vi "校准信息转u16数组.vi"(11 "关键参数":T1(array[cluster])) -> (3 "添加的数组":u16[](array[numeric]))   [LabVIEW 2016, in "MB SLAVE.lvlib"]
uses:
  MB SLAVE.lvlib
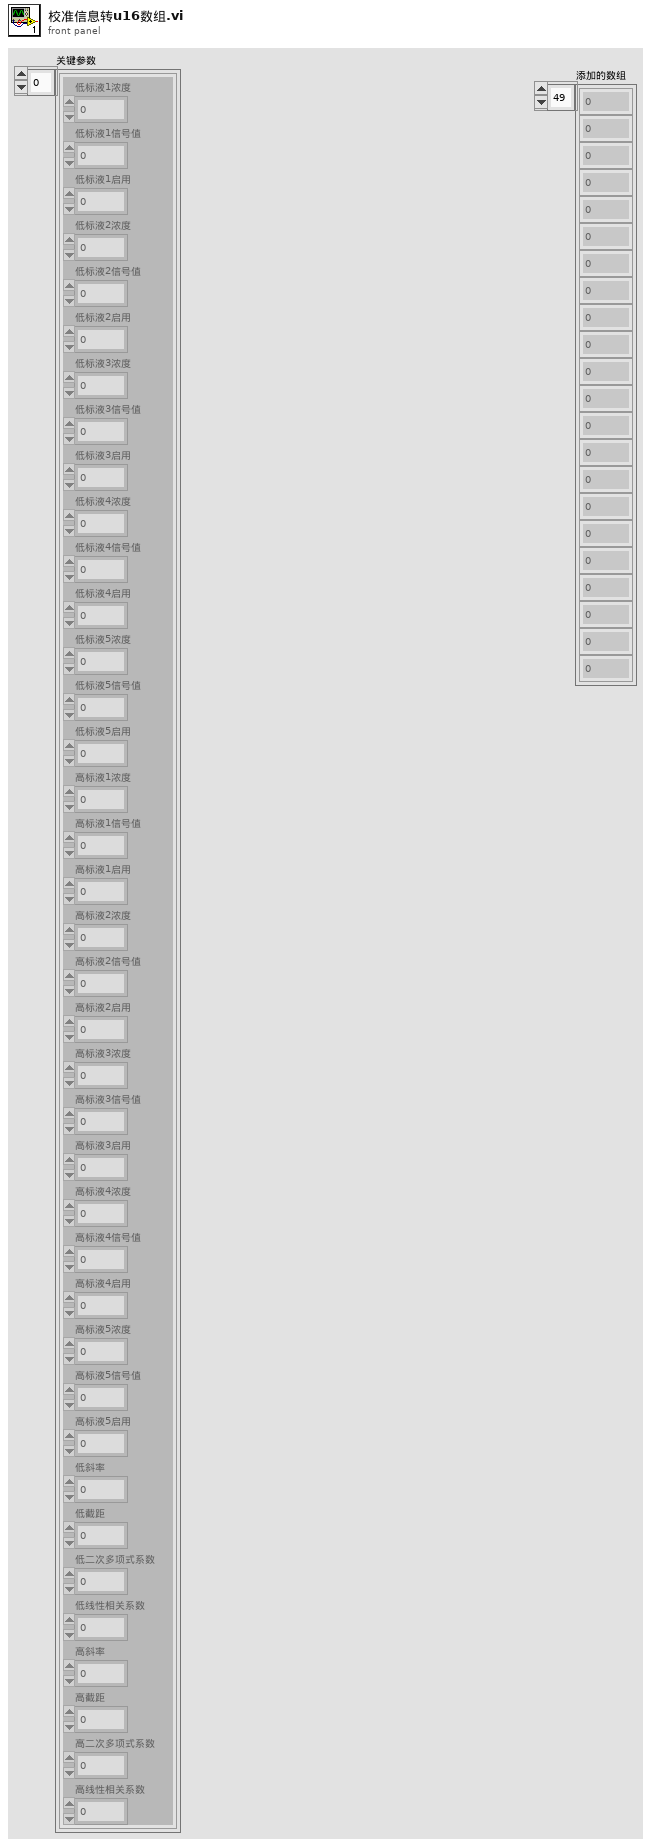
[diagram p1: front panel]
types:
  T1 = cluster{"低标液1浓度":dbl, "低标液1信号值":dbl, "低标液1启用":u16, "低标液2浓度":dbl, "低标液2信号值":dbl, "低标液2启用":u16, "低标液3浓度":dbl, "低标液3信号值":dbl, "低标液3启用":u16, "低标液4浓度":dbl, "低标液4信号值":dbl, "低标液4启用":u16, "低标液5浓度":dbl, "低标液5信号值":dbl, "低标液5启用":u16, "高标液1浓度":dbl, "高标液1信号值":dbl, "高标液1启用":u16, "高标液2浓度":dbl, "高标液2信号值":dbl, "高标液2启用":u16, "高标液3浓度":dbl, "高标液3信号值":dbl, "高标液3启用":u16, "高标液4浓度":dbl, "高标液4信号值":dbl, "高标液4启用":u16, "高标液5浓度":dbl, "高标液5信号值":dbl, "高标液5启用":u16, "低斜率":dbl, "低截距":dbl, "低二次多项式系数":dbl, "低线性相关系数":dbl, "高斜率":dbl, "高截距":dbl, "高二次多项式系数":dbl, "高线性相关系数":dbl}[]
  T2 = cluster{"低标液1浓度":dbl, "低标液1信号值":dbl, "低标液1启用":u16, "低标液2浓度":dbl, "低标液2信号值":dbl, "低标液2启用":u16, "低标液3浓度":dbl, "低标液3信号值":dbl, "低标液3启用":u16, "低标液4浓度":dbl, "低标液4信号值":dbl, "低标液4启用":u16, "低标液5浓度":dbl, "低标液5信号值":dbl, "低标液5启用":u16, "高标液1浓度":dbl, "高标液1信号值":dbl, "高标液1启用":u16, "高标液2浓度":dbl, "高标液2信号值":dbl, "高标液2启用":u16, "高标液3浓度":dbl, "高标液3信号值":dbl, "高标液3启用":u16, "高标液4浓度":dbl, "高标液4信号值":dbl, "高标液4启用":u16, "高标液5浓度":dbl, "高标液5信号值":dbl, "高标液5启用":u16, "低斜率":dbl, "低截距":dbl, "低二次多项式系数":dbl, "低线性相关系数":dbl, "高斜率":dbl, "高截距":dbl, "高二次多项式系数":dbl, "高线性相关系数":dbl}
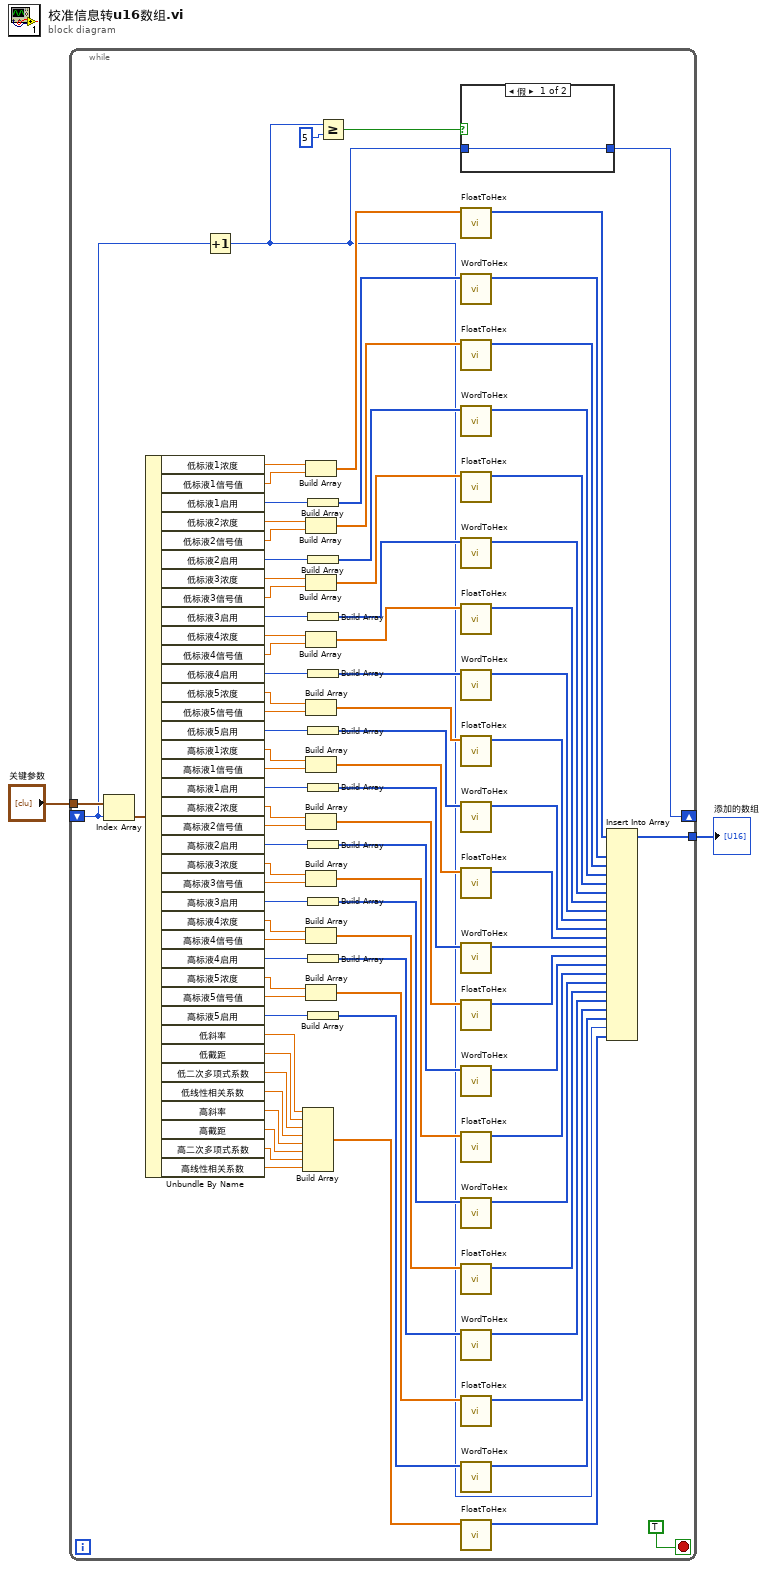
[diagram p0: block diagram]
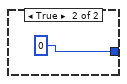
[diagram p2: hidden frame]
diagram:
  n1 = while {
    tunnel: "关键参数" -> [w90]
    shift-right: [w83] -> _
    shift-left: _ -> [w87]
    tunnel: [w86] -> w1
    stop <- TRUE stop-if-true
    n2 = Index Array(array=w90, index=w87) -> (element=w89:T2)
    n3 = Unbundle By Name(w89) -> ("低标液1浓度"=w82:dbl, "低标液1信号值"=w81:dbl, "低标液1启用"=w78:u16, "低标液2浓度"=w75:dbl, "低标液2信号值"=w74:dbl, "低标液2启用"=w91:u16, "低标液3浓度"=w68:dbl, "低标液3信号值"=w67:dbl, "低标液3启用"=w66:u16, "低标液4浓度"=w60:dbl, "低标液4信号值"=w59:dbl, "低标液4启用"=w58:u16, "低标液5浓度"=w53:dbl, "低标液5信号值"=w52:dbl, "低标液5启用"=w51:u16, "高标液1浓度"=w46:dbl, "高标液1信号值"=w45:dbl, "高标液1启用"=w43:u16, "高标液2浓度"=w39:dbl, "高标液2信号值"=w38:dbl, "高标液2启用"=w37:u16, "高标液3浓度"=w30:dbl, "高标液3信号值"=w29:dbl, "高标液3启用"=w28:u16, "高标液4浓度"=w23:dbl, "高标液4信号值"=w22:dbl, "高标液4启用"=w21:u16, "高标液5浓度"=w20:dbl, "高标液5信号值"=w19:dbl, "高标液5启用"=w18:u16, "低斜率"=w12:dbl, "低截距"=w11:dbl, "低二次多项式系数"=w10:dbl, "低线性相关系数"=w9:dbl, "高斜率"=w8:dbl, "高截距"=w7:dbl, "高二次多项式系数"=w6:dbl, "高线性相关系数"=w5:dbl)
    n4 = Increment(x=w87) -> (x+1=w13:u16)
    n5 = Build Array(w12, w11, w10, w9, w8, w7, w6, w5) -> (w4:dbl[])
    n6 = Build Array(w82, w81) -> (w80:dbl[])
    n7 = Build Array(w75, w74) -> (w73:dbl[])
    n8 = Build Array(w68, w67) -> (w69:dbl[])
    n9 = Build Array(w60, w59) -> (w62:dbl[])
    n10 = Build Array(w53, w52) -> (w55:dbl[])
    n11 = Build Array(w46, w45) -> (w48:dbl[])
    n12 = Build Array(w39, w38) -> (w41:dbl[])
    n13 = Build Array(w30, w29) -> (w34:dbl[])
    n14 = Build Array(w23, w22) -> (w32:dbl[])
    n15 = Build Array(w20, w19) -> (w25:dbl[])
    n16 = Build Array(w78) -> (w77:u16[])
    n17 = Build Array(w91) -> (w72:u16[])
    n18 = Build Array(w66) -> (w65:u16[])
    n19 = Build Array(w58) -> (w61:u16[])
    n20 = Build Array(w51) -> (w54:u16[])
    n21 = Build Array(w43) -> (w47:u16[])
    n22 = Build Array(w37) -> (w40:u16[])
    n23 = Build Array(w28) -> (w33:u16[])
    n24 = Build Array(w21) -> (w31:u16[])
    n25 = Build Array(w18) -> (w24:u16[])
    n26 = Greater Or Equal?(x=w13, y=u16 5) -> (x >= y?=w84:bool)
    n27 = case shown="假" w84 {
      tunnel: [w92 u16 0] -> w83
      tunnel: w13 -> [w92 _]
      frame False {
      }
      frame True {
      }
    }
    n28 = call "FloatToHex.vi"("FLOAT"=w80) -> ("交织的数组"=w79:u16[])  [unwired: 10 in]
    n29 = call "WordToHex.vi"("WORD"=w77) -> ("数组"=w76:u16[])  [unwired: 10 in]
    n30 = call "FloatToHex.vi"("FLOAT"=w73) -> ("交织的数组"=w71:u16[])  [unwired: 10 in]
    n31 = call "WordToHex.vi"("WORD"=w72) -> ("数组"=w70:u16[])  [unwired: 10 in]
    n32 = call "FloatToHex.vi"("FLOAT"=w69) -> ("交织的数组"=w64:u16[])  [unwired: 10 in]
    n33 = call "WordToHex.vi"("WORD"=w65) -> ("数组"=w63:u16[])  [unwired: 10 in]
    n34 = call "FloatToHex.vi"("FLOAT"=w62) -> ("交织的数组"=w57:u16[])  [unwired: 10 in]
    n35 = call "WordToHex.vi"("WORD"=w61) -> ("数组"=w56:u16[])  [unwired: 10 in]
    n36 = call "FloatToHex.vi"("FLOAT"=w55) -> ("交织的数组"=w50:u16[])  [unwired: 10 in]
    n37 = call "WordToHex.vi"("WORD"=w54) -> ("数组"=w49:u16[])  [unwired: 10 in]
    n38 = call "FloatToHex.vi"("FLOAT"=w48) -> ("交织的数组"=w44:u16[])  [unwired: 10 in]
    n39 = call "WordToHex.vi"("WORD"=w47) -> ("数组"=w42:u16[])  [unwired: 10 in]
    n40 = call "FloatToHex.vi"("FLOAT"=w41) -> ("交织的数组"=w36:u16[])  [unwired: 10 in]
    n41 = call "WordToHex.vi"("WORD"=w40) -> ("数组"=w35:u16[])  [unwired: 10 in]
    n42 = call "FloatToHex.vi"("FLOAT"=w34) -> ("交织的数组"=w27:u16[])  [unwired: 10 in]
    n43 = call "WordToHex.vi"("WORD"=w33) -> ("数组"=w26:u16[])  [unwired: 10 in]
    n44 = call "FloatToHex.vi"("FLOAT"=w32) -> ("交织的数组"=w17:u16[])  [unwired: 10 in]
    n45 = call "WordToHex.vi"("WORD"=w31) -> ("数组"=w16:u16[])  [unwired: 10 in]
    n46 = call "FloatToHex.vi"("FLOAT"=w25) -> ("交织的数组"=w15:u16[])  [unwired: 10 in]
    n47 = call "WordToHex.vi"("WORD"=w24) -> ("数组"=w14:u16[])  [unwired: 10 in]
    n48 = call "FloatToHex.vi"("FLOAT"=w4) -> ("交织的数组"=w3:u16[])  [unwired: 10 in]
    n49 = Insert Into Array(array=w79, new element #1=w76, new element #2=w71, new element #3=w70, new element #4=w64, new element #5=w63, new element #6=w57, new element #7=w56, new element #8=w50, new element #9=w49, new element #10=w44, new element #11=w42, new element #12=w36, new element #13=w35, new element #14=w27, new element #15=w26, new element #16=w17, new element #17=w16, new element #18=w15, new element #19=w14, new element #20=w13, new element #21=w3) -> (w86:u16[])  [unwired: 1 in]
  }
  "添加的数组" <- w1
